vi "Requester.vi"(8 "error in":errorcluster) -> (0 "error out":errorcluster)   [LabVIEW 2024]
uses:
  NATS Client/NATS Client.lvclass/NATS Client.ctl
  <vilib>/NATS/NATS Core/VIs/NATS CLOSE.vi
  NATS Client/get async stop notifier.vi
  NATS Client/Get Connection DVR.vi
  NATS Client/get subscriptions queue.vi
  NATS Client/Get subscription map.vi
  NATS Client/Get error queue.vi
  NATS Subscription/NATS Subscription.lvclass
  NATS Client/NATS Client.lvclass
panel:
  out "Response Payload":string
  in  "Request Payload":string="update me to see a request response"
  out "loop error":errorcluster
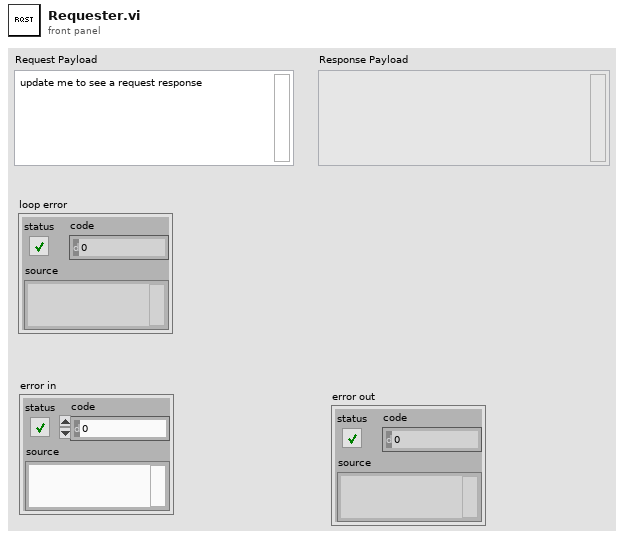
[diagram p1: front panel]
types:
  T1 = typedef "NATS Core.lvlib/nats message.ctl" = cluster{"subject":string, "payload":string, "sub id":string, "reply-to":string, "headers":string, "type":T2, "received":timestamp}
  T2 = typedef "NATS Core.lvlib/msg type.ctl" = enum16{"Undefined", "MSG", "HMSG", "+OK", "PING", "PONG", "-ERR", "INFO"}
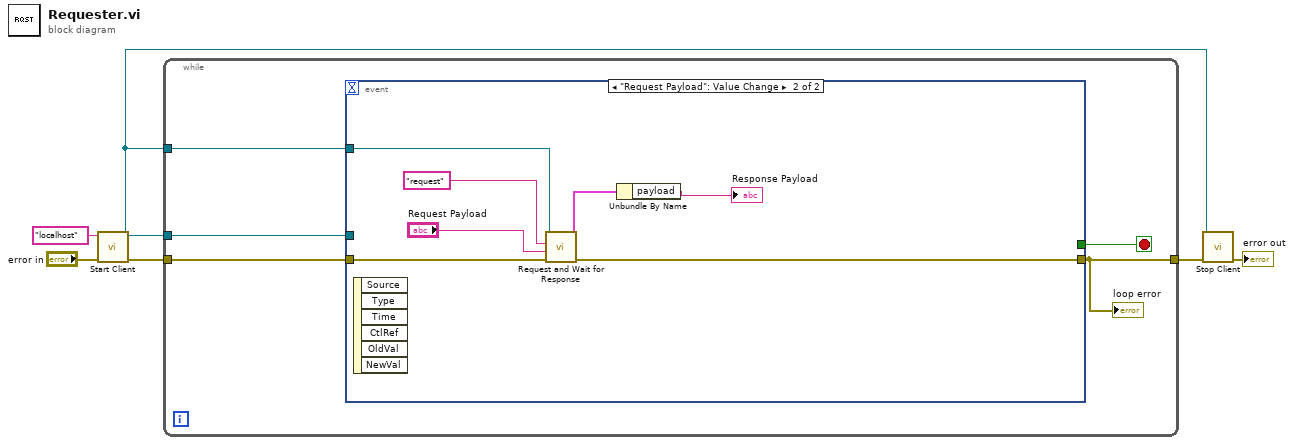
[diagram p0: block diagram]
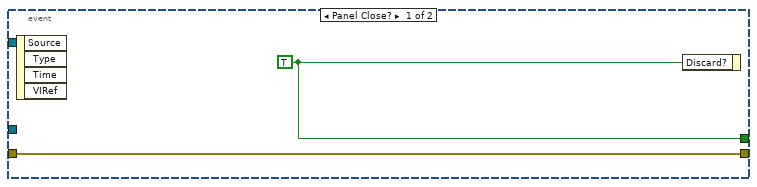
[diagram p2: hidden frame]
diagram:
  n1 = call "Start Client.vi"("error in"="error in", "address"="localhost") -> ("error out"=w6:errorcluster, "NATS Client out"=w3:refnum<class "NATS Client.lvclass">)  [unwired: 8 in]
  n2 = while {
    tunnel: w3 -> [w9]
    tunnel: w3 -> [w8]
    tunnel: w6 -> [w10]
    tunnel: [w7] -> w4
    stop <- w11 stop-if-true
    n3 = event shown="[1] \"Request Payload\": Value Change" {
      selector: _ -> [_ _]
      dyn-events: _ -> [_ _]
      timeout: _ -> [_ _]
      tunnel: [w13 _] -> w11
      tunnel: w10 -> [w12 w20]
      tunnel: [w12 w16] -> w7
      tunnel: w9 -> [_ _]
      tunnel: w8 -> [_ w19]
      event Panel Close? {
        w13 = TRUE ("Discard?")
        n4 = event-data() -> ()  [unwired: 1 in, 4 out]
        n5 = event-data("Discard?"=w13) -> ()  [unwired: 1 in, 1 out]
      }
      event "Request Payload": Value Change {
        n6 = event-data() -> ()  [unwired: 1 in, 6 out]
        n7 = call "Request and Wait for Response.vi"("error in"=w20, "payload"="Request Payload", "subject"="request" ("Subject"), "NATS Client in"=w19) -> ("error out"=w16:errorcluster, "nats message"=w15:T1)  [unwired: 5 in, 1 out]
        n8 = Unbundle By Name(w15) -> ("payload"=→"Response Payload":string)
      }
    }
    "loop error" <- w7
  }
  n9 = call "Stop Client.vi"("error in"=w4, "NATS Client"=w3) -> ("error out"=→"error out":errorcluster)  [unwired: 9 in]
